vi "Build Tree Data Type.vi"(4 "Tag Blacklist":i8[](array[numeric]), 6 "Show IDs (True)":bool=TRUE, 7 "Test ID":string, 8 "error in (no error)":errorcluster, 11 "Test Executive in":refnum<class "Test Executive.lvclass">) -> (0 "error out":errorcluster, 2 "Tree Data":T1(array[cluster]), 3 "Test Executive out":refnum<class "Test Executive.lvclass">)   [LabVIEW 2020, in "Test Executive.lvlib" / "Test Executive.lvclass"]
uses:
  <vilib>/gpm_packages/@cs/test-executive/Source/Test Executive/TestExecutive/Test Executive.lvclass
  <vilib>/gpm_packages/@cs/test-executive/Source/Test Executive/TestExecutive/Test Executive.lvclass/Test Executive.ctl
  <vilib>/gpm_packages/@cs/linked-list/Source/Linked List/Linked List Ref/Linked List Ref.lvclass
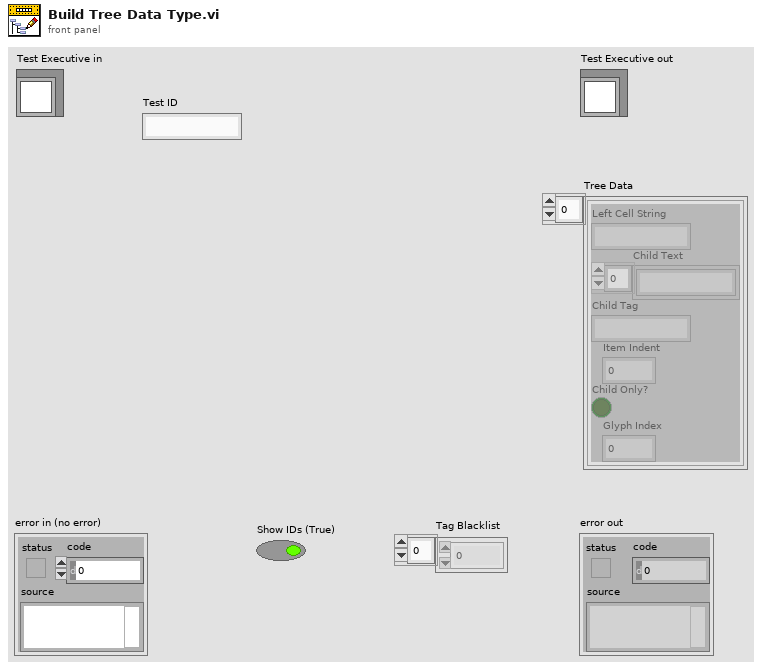
[diagram p1: front panel]
types:
  T1 = cluster{"Left Cell String":string, "Child Text":string[], "Child Tag":string, "Item Indent":i32, "Child Only?":bool, "Glyph Index":i32}[]
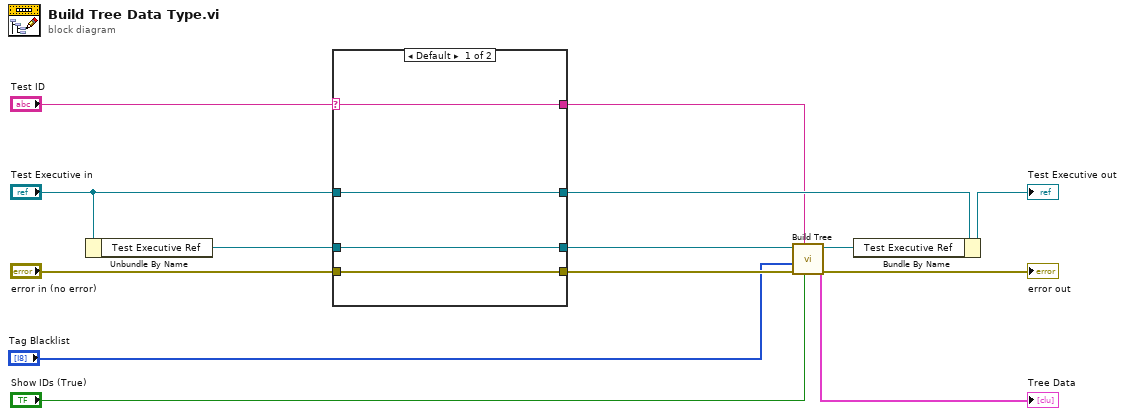
[diagram p0: block diagram]
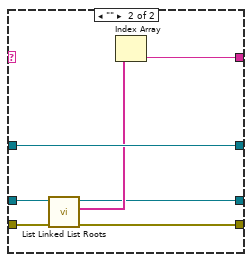
[diagram p2: hidden frame]
diagram:
  n1 = Unbundle By Name("Test Executive in") -> ("Test Executive Ref"=w7:refnum<data-value>)
  n2 = case shown="Default" "Test ID" {
    selector: "Test ID" -> [w17 _]
    tunnel: "Test Executive in" -> [w18 w25]
    tunnel: w7 -> [w16 w24]
    tunnel: [w18 w25] -> w8
    tunnel: "error in (no error)" -> [w15 w23]
    tunnel: [w17 w21] -> w2
    tunnel: [w16 w20] -> w6
    tunnel: [w15 w19] -> w4
    frame Default {
    }
    frame "" {
      n3 = call <vilib>:"List Linked List Roots.vi"("error in (no error)"=w23, "Linked List Ref"=w24) -> ("error out"=w19:errorcluster, "Root IDs"=w22:string[], "Linked List Ref out"=w20:refnum<data-value>)  [unwired: 6 in, 1 out]
      n4 = Index Array(array=w22) -> (element=w21:string)  [unwired: 1 in]
    }
  }
  n5 = call <vilib>:"Build Tree.vi"("Show IDs"="Show IDs (True)", "Linked List ID"=w2, "error in (no error)"=w4, "Tag Blacklist"="Tag Blacklist", "Linked List Ref"=w6) -> ("error out"=→"error out":errorcluster, "Tree Data"=→"Tree Data":T1, "Linked List Ref out"=w12:refnum<data-value>)  [unwired: 4 in]
  n6 = Bundle By Name(cluster=w8, "Test Executive Ref"=w12) -> (→"Test Executive out":refnum<class "Test Executive.lvclass">)
